vi "Check parts acceptable - toplayer.vi"(6 "Stack IDs":string[](array[string]), 7 "DB out stack":string[][](array[string]), 8 "error in (no error)":errorcluster, 9 "Toplayer IDs":string[](array[string]), 10 "DB out top":string[][](array[string]), 11 "Database Entry in":refnum<class "Database Entry.lvclass">) -> (0 "error out":errorcluster, 2 "Replace parts out":bool, 3 "Database Entry out":refnum<class "Database Entry.lvclass">, 4 "Abort?":bool)   [LabVIEW 2021, in "Database Entry.lvclass"]
uses:
  Database Entry.lvclass
panel:
  in  "Database out - stack":i32[](listbox)
  in  "Replace parts top":bool
  in  "Are these parts satisfactory?":bool
  in  "Abort":bool
  in  "Submit":bool
  in  "Database out - toplayer":i32[](listbox)
  # "(If parts are satisfactory, this assembly run will be written into Postgres.)"
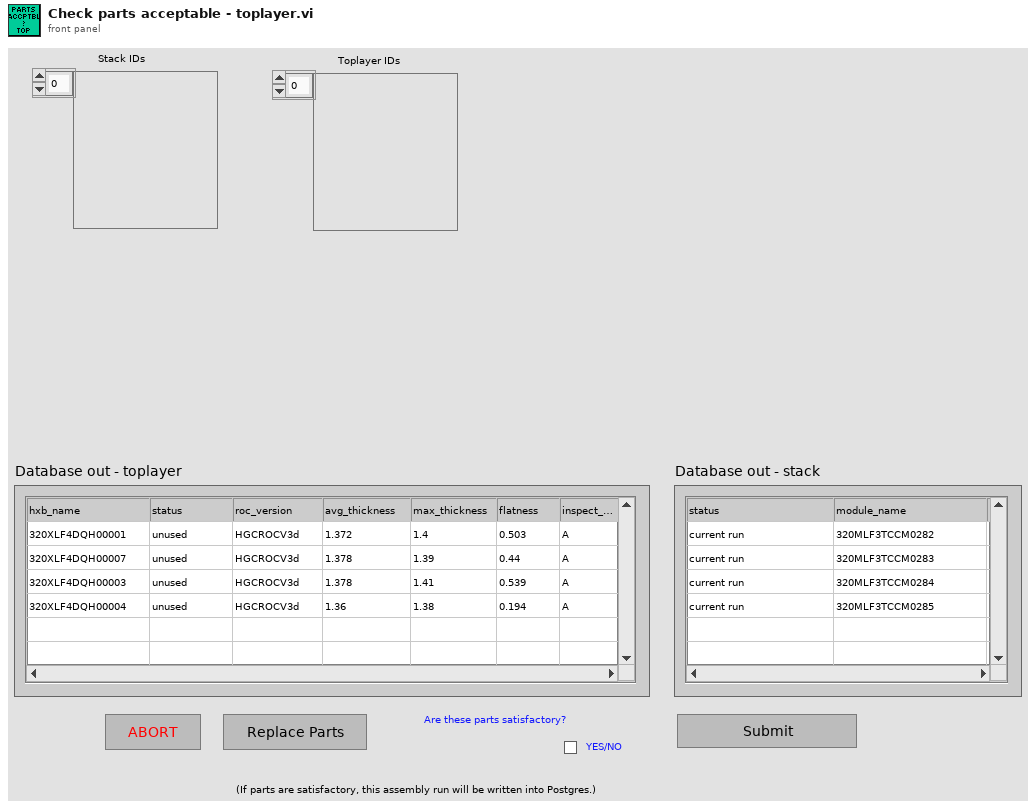
[diagram p1: front panel]
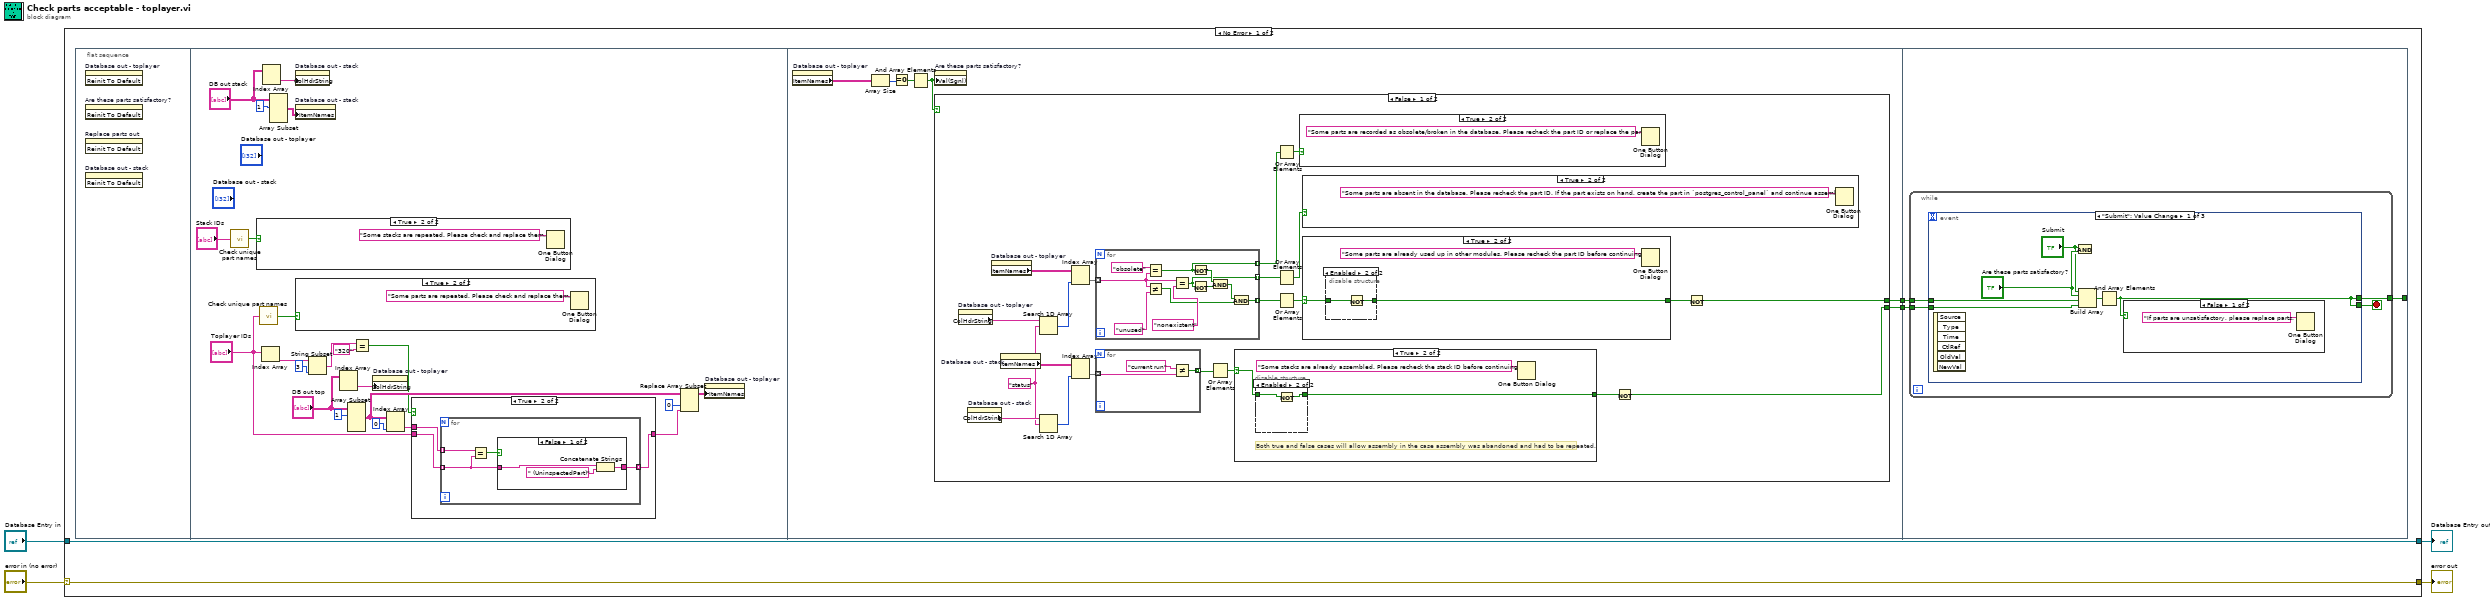
[diagram p0: block diagram]
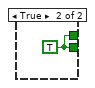
[diagram p12: hidden frame]
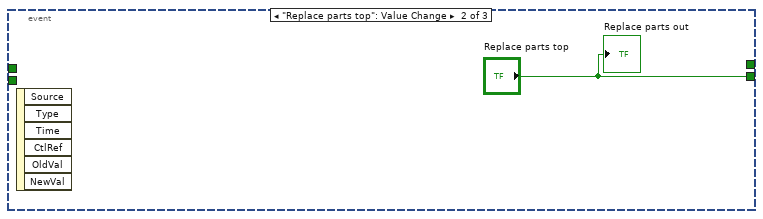
[diagram p14: hidden frame]
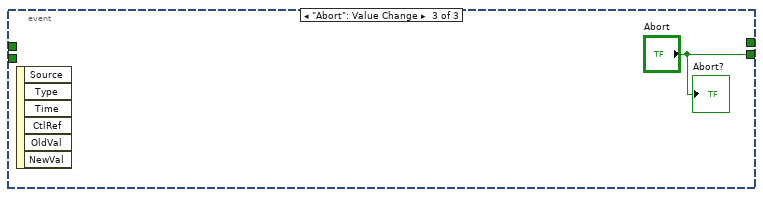
[diagram p15: hidden frame]
diagram:
  n1 = case shown="No Error" "error in (no error)" {
    selector: "error in (no error)" -> [w8 w120]
    tunnel: [w8 w120] -> w3
    tunnel: [w7 w119] -> w1
    tunnel: "Database Entry in" -> [w7 w119]
    frame No Error {
      n2 = flat-sequence {
        tunnel: [w46] -> w6
        tunnel: [w45] -> w5
        tunnel: [w105] -> _
        tunnel: w6 -> [w104]
        tunnel: w5 -> [w103]
        frame #0 {
          n3 = invoke on="Database out - toplayer" class="MCListbox (strict)" method="Reinit To Default"() -> ()  [unwired: 3 in, 3 out]
          n4 = invoke on="Are these parts satisfactory?" class="Bool (strict)" method="Reinit To Default"() -> ()  [unwired: 3 in, 3 out]
          n5 = invoke on="Replace parts out" class="Bool (strict)" method="Reinit To Default"() -> ()  [unwired: 3 in, 3 out]
          n6 = invoke on="Database out - stack" class="MCListbox (strict)" method="Reinit To Default"() -> ()  [unwired: 3 in, 3 out]
        }
        frame #1 {
          n7 = call "Check unique part names.vi"("Part IDs"="Stack IDs") -> ("Parts repeated"=w13:bool)
          n8 = case shown="True" w13 {
            frame False {
            }
            frame True {
              n9 = One Button Dialog(message="Some stacks are repeated. Please check and replace them.") -> ()  [unwired: 1 in, 1 out]
            }
          }
          n10 = call "Check unique part names.vi"("Part IDs"="Toplayer IDs") -> ("Parts repeated"=w15:bool)
          n11 = Index Array(array="Toplayer IDs") -> (element=w21:string)  [unwired: 1 in]
          n12 = Index Array(array="DB out stack") -> (element=w12:string[])  [unwired: 2 in]
          n13 = Array Subset(array="DB out stack", index (row)=1 ("index")) -> (w10:string[][])  [unwired: 3 in]
          n14 = property on="Database out - stack" class="MCListbox (strict)"("ColHdrString"=w12) -> ()  [unwired: 2 in, 2 out]
          n15 = property on="Database out - stack" class="MCListbox (strict)"("ItemNames"=w10) -> ()  [unwired: 2 in, 2 out]
          n16 = case shown="True" w15 {
            frame False {
            }
            frame True {
              n17 = One Button Dialog(message="Some parts are repeated. Please check and replace them.") -> ()  [unwired: 1 in, 1 out]
            }
          }
          n18 = String Subset(string=w21, length (rest)=3 ("length (rest)")) -> (substring=w17:string)  [unwired: 1 in]
          n19 = Index Array(array="DB out top") -> (element=w23:string[])  [unwired: 2 in]
          n20 = Array Subset(array="DB out top", index (row)=1 ("index")) -> (w27:string[][])  [unwired: 3 in]
          n21 = Equal?(x=w17, y="320") -> (x = y?=w19:bool)
          n22 = property on="Database out - toplayer" class="MCListbox (strict)"("ColHdrString"=w23) -> ()  [unwired: 2 in, 2 out]
          n23 = Index Array(array=w27, index (col)=0 ("disabled index (col)")) -> (element=w28:string[])  [unwired: 1 in]
          n24 = case shown="True" w19 {
            tunnel: w28 -> [_ w36]
            tunnel: [w33 w35] -> w25
            tunnel: "Toplayer IDs" -> [w33 w34]
            frame False {
            }
            frame True {
              n25 = for {
                tunnel: w36 -> [w39] mode=indexing
                tunnel: w34 -> [w37] mode=indexing
                tunnel: [w38] -> w35 mode=indexing
                n26 = Equal?(x=w39, y=w37) -> (x = y?=w40:bool)
                n27 = case shown="False" w40 {
                  tunnel: w37 -> [w43 w44]
                  tunnel: [w41 w44] -> w38
                  frame False {
                    n28 = Concatenate Strings(w43, " (UninspectedPart)" ("string")) -> (w41:string)
                  }
                  frame True {
                  }
                }
              }
            }
          }
          n29 = Replace Array Subset(array=w27, new element=w25, index (col)=0 ("disabled index (col)")) -> (w22:string[][])  [unwired: 1 in]
          n30 = property on="Database out - toplayer" class="MCListbox (strict)"("ItemNames"=w22) -> ()  [unwired: 2 in, 2 out]
        }
        frame #2 {
          n31 = property on="Database out - toplayer" class="MCListbox (strict)"() -> ("ItemNames"=w48:string[][])  [unwired: 2 in, 2 out]
          n32 = Array Size(array=w48) -> (size(s)=w49:i32[])
          n33 = Equal To 0?(x=w49) -> (x = 0?=w50:bool[])
          n34 = And Array Elements(Boolean array=w50) -> (logical AND=w47:bool)
          n35 = property on="Are these parts satisfactory?" class="Bool (strict)"("Val(Sgnl)"=w47) -> ()  [unwired: 2 in, 2 out]
          n36 = case shown="False" w47 {
            tunnel: [w59 w102] -> w46
            tunnel: [w57 w102] -> w45
            frame False {
              w64 = "status" ("element")
              n37 = property on="Database out - toplayer" class="MCListbox (strict)"() -> ("ColHdrString"=w70:string[])  [unwired: 2 in, 2 out]
              n38 = property on="Database out - stack" class="MCListbox (strict)"() -> ("ColHdrString"=w65:string[])  [unwired: 2 in, 2 out]
              n39 = property on="Database out - toplayer" class="MCListbox (strict)"() -> ("ItemNames"=w71:string[][])  [unwired: 2 in, 2 out]
              n40 = property on="Database out - stack" class="MCListbox (strict)"() -> ("ItemNames"=w63:string[][])  [unwired: 2 in, 2 out]
              n41 = Search 1D Array(1D array=w70, element=w64) -> (index of element=w55:i32)  [unwired: 1 in]
              n42 = Search 1D Array(1D array=w65, element=w64) -> (index of element=w53:i32)  [unwired: 1 in]
              n43 = Index Array(array=w71, index (col)=w55) -> (element=w56:string[])  [unwired: 1 in]
              n44 = Index Array(array=w63, index (col)=w53) -> (element=w54:string[])  [unwired: 1 in]
              n45 = for {
                tunnel: w56 -> [w96] mode=indexing
                tunnel: [w98] -> w69 mode=indexing
                tunnel: [w92] -> w68 mode=indexing
                tunnel: [w93] -> w52 mode=indexing
                n46 = Equal?(x="obsolete" ("y"), y=w96) -> (x = y?=w93:bool)
                n47 = Not Equal?(x=w96, y="unused") -> (x != y?=w99:bool)
                n48 = Equal?(x=w96, y="nonexistent") -> (x = y?=w92:bool)
                n49 = Not(x=w93) -> (.not. x?=w95:bool)
                n50 = Not(x=w92) -> (.not. x?=w94:bool)
                n51 = And(x=w95, y=w94) -> (x .and. y?=w91:bool)
                n52 = And(x=w91, y=w99) -> (x .and. y?=w98:bool)
              }
              n53 = for {
                tunnel: w54 -> [w82] mode=indexing
                tunnel: [w81] -> w62 mode=indexing
                n54 = Not Equal?(x="current run" ("y"), y=w82) -> (x != y?=w81:bool)
              }
              n55 = Or Array Elements(Boolean array=w62) -> (logical OR=w61:bool)
              n56 = case shown="True" w61 {
                selector: w61 -> [w73 w75]
                tunnel: [w73 w74] -> w58
                frame False {
                }
                frame True {
                  # "Both true and false cases will allow assembly in the case assembly was abandoned and had to be repeated."
                  n57 = disable-structure shown="Enabled" {
                    disable-tunnel: w75 -> [w77 w79]
                    disable-tunnel: [w77 w78] -> w74
                    frame Disabled {
                    }
                    frame Enabled {
                      n58 = Not(x=w79) -> (.not. x?=w78:bool)
                    }
                  }
                  n59 = One Button Dialog(message="Some stacks are already assembled. Please recheck the stack ID before continuing.") -> ()  [unwired: 1 in, 1 out]
                }
              }
              n60 = Or Array Elements(Boolean array=w52) -> (logical OR=w51:bool)
              n61 = Or Array Elements(Boolean array=w68) -> (logical OR=w67:bool)
              n62 = Or Array Elements(Boolean array=w69) -> (logical OR=w66:bool)
              n63 = case shown="True" w51 {
                frame False {
                }
                frame True {
                  n64 = One Button Dialog(message="Some parts are recorded as obsolete/broken in the database. Please recheck the part ID or replace the part.") -> ()  [unwired: 1 in, 1 out]
                }
              }
              n65 = case shown="True" w67 {
                frame False {
                }
                frame True {
                  n66 = One Button Dialog(message="Some parts are absent in the database. Please recheck the part ID. If the part exists on hand, create the part in `postgres_control_panel` and continue assembly. ") -> ()  [unwired: 1 in, 1 out]
                }
              }
              n67 = case shown="True" w66 {
                selector: w66 -> [w83 w85]
                tunnel: [w83 w84] -> w60
                frame False {
                }
                frame True {
                  n68 = disable-structure shown="Enabled" {
                    disable-tunnel: w85 -> [w87 w89]
                    disable-tunnel: [w87 w88] -> w84
                    frame Disabled {
                    }
                    frame Enabled {
                      n69 = Not(x=w89) -> (.not. x?=w88:bool)
                    }
                  }
                  n70 = One Button Dialog(message="Some parts are already used up in other modules. Please recheck the part ID before continuing.") -> ()  [unwired: 1 in, 1 out]
                }
              }
              n71 = Not(x=w58) -> (.not. x?=w57:bool)
              n72 = Not(x=w60) -> (.not. x?=w59:bool)
            }
            frame True {
              w102 = TRUE
            }
          }
        }
        frame #3 {
          n73 = while {
            tunnel: [w108] -> w105
            tunnel: w104 -> [w107]
            tunnel: w103 -> [w106]
            stop <- w109 stop-if-true
            n74 = event shown="[0] \"Submit\": Value Change" {
              selector: _ -> [_ _ _]
              dyn-events: _ -> [_ _ _]
              timeout: _ -> [_ _ _]
              tunnel: [w110 "Replace parts top" "Abort"] -> w109
              tunnel: [w110 _ _] -> w108
              tunnel: w107 -> [w113 _ _]
              tunnel: w106 -> [w112 _ _]
              event "Submit": Value Change {
                n75 = event-data() -> ()  [unwired: 1 in, 6 out]
                n76 = And(x="Submit", y="Are these parts satisfactory?") -> ()  [unwired: 1 out]
                n77 = Build Array("Submit", "Are these parts satisfactory?", w113, w112) -> (w111:bool[])
                n78 = And Array Elements(Boolean array=w111) -> (logical AND=w110:bool)
                n79 = case shown="False" w110 {
                  frame False {
                    n80 = One Button Dialog(message="If parts are unsatisfactory, please replace parts. ") -> ()  [unwired: 1 in, 1 out]
                  }
                  frame True {
                  }
                }
              }
              event "Replace parts top": Value Change {
                n81 = event-data() -> ()  [unwired: 1 in, 6 out]
                "Replace parts out" <- "Replace parts top"
              }
              event "Abort": Value Change {
                n82 = event-data() -> ()  [unwired: 1 in, 6 out]
                "Abort?" <- "Abort"
              }
            }
          }
        }
      }
    }
    frame Error {
    }
  }
  "error out" <- w3
  "Database Entry out" <- w1
